vi "xeva-checkTime.vi"(3 "error in (no error)":errorcluster, 4 "xeva-time":dbl, 5 "xeva-camref":T1) -> (0 "error out":errorcluster, 1 "xeva-time-ok":bool)   [LabVIEW 2015]
uses:
  <vilib>/Xenics Infrared Solutions/Xeneth LabVIEW API/VIs/Controls/Camara.ctl
  <vilib>/Xenics Infrared Solutions/Xeneth LabVIEW API/Xeneth.lvlib
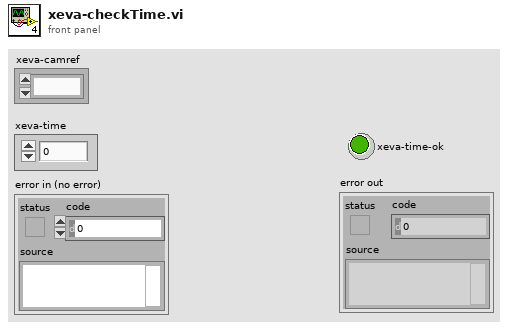
[diagram p1: front panel]
types:
  T1 = typedef "Xeneth.lvlib/Camara.ctl" = refnum<k1>
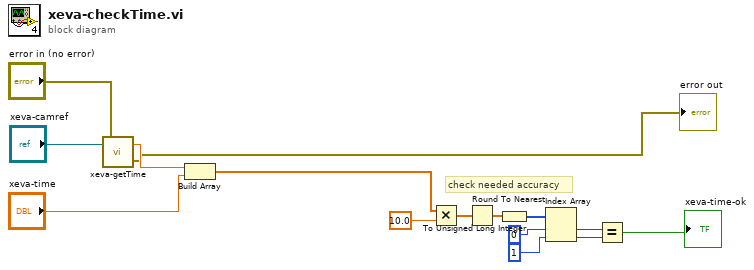
[diagram p0: block diagram]
diagram:
  # "check needed accuracy"
  n1 = call "xeva-getTime.vi"("error in (no error)"="error in (no error)", "xeva-camref"="xeva-camref") -> ("error out"=→"error out":errorcluster, "xeva-time"=w11:dbl)
  n2 = Build Array(w11, "xeva-time") -> (w9:dbl[])
  n3 = Multiply(x=w9, y=10.0) -> (x*y=w12:dbl[])
  n4 = Round To Nearest(number=w12) -> (nearest integer value=w8:dbl[])
  n5 = To Unsigned Long Integer(number=w8) -> (unsigned 32bit integer=w7:u32[])
  n6 = Index Array(array=w7, index #1=0 ("index"), index #2=1 ("index")) -> (element #1=w3:u32, element #2=w4:u32)
  n7 = Equal?(x=w3, y=w4) -> (x = y?=→"xeva-time-ok":bool)
